vi "Set Sample.vi"(8 "error in (no error)":errorcluster, 10 "Sample":refnum<class "Sample.lvclass">, 11 "He Line in":refnum<class "He Line.lvclass">) -> (0 "error out":errorcluster, 1 "overflow?":bool, 2 "overflow Sample":refnum<class "Sample.lvclass">, 3 "He Line out":refnum<class "He Line.lvclass">)   [LabVIEW 2015, in "cRIO-Carbondioxide.lvlib" / "CO2-Actor.lvlib" / "He Line.lvclass"]
uses:
  He Line.lvclass
  subs/Sample/Sample.lvclass
  He Line.lvclass/He Line.ctl
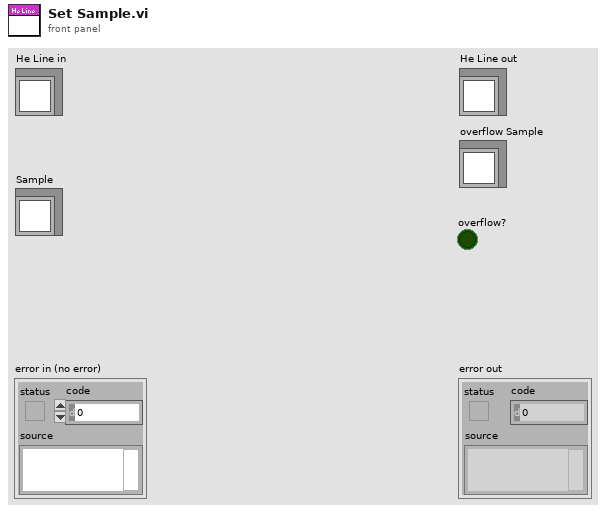
[diagram p1: front panel]
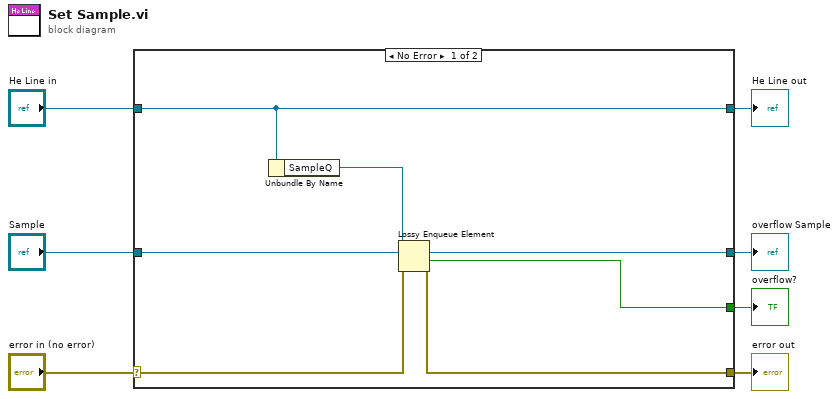
[diagram p0: block diagram]
diagram:
  n1 = case shown="No Error" "error in (no error)" {
    selector: "error in (no error)" -> [w12 w16]
    tunnel: [w11 w16] -> w6
    tunnel: [w14 w15] -> w4
    tunnel: "He Line in" -> [w14 w15]
    tunnel: "Sample" -> [w10 _]
    tunnel: [w9 _] -> w2
    tunnel: [w8 _] -> w1
    frame No Error {
      n2 = Unbundle By Name(w14) -> ("SampleQ"=w13:refnum<queue>)
      n3 = Lossy Enqueue Element(queue=w13, element=w10, error in (no error)=w12) -> (overflow element=w9:refnum<class "Sample.lvclass">, overflow?=w8:bool, error out=w11:errorcluster)  [unwired: 1 out]
    }
    frame Error {
    }
  }
  "error out" <- w6
  "He Line out" <- w4
  "overflow Sample" <- w2
  "overflow?" <- w1
